vi "PostBuild.vi"(8 "error in (no error)":errorcluster, 9 "GeneratedFiles in":path[](array[path]), 10 "GeneratedDirectories in":path[](array[path]), 11 "Build in":refnum<class "AB_Build.lvclass">) -> (0 "error out":errorcluster, 1 "GeneratedFiles out":path[](array[path]), 2 "GeneratedDirectories out":path[](array[path]), 3 "Build out":refnum<class "AB_Build.lvclass">)   [LabVIEW 2020, in "AB_Build.lvclass"]
uses:
  <vilib>/AppBuilder/AB_Classes/Build/AB_Build.lvclass
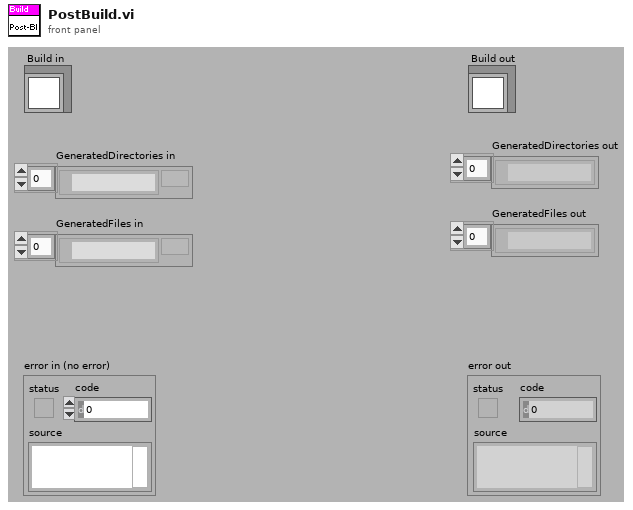
[diagram p1: front panel]
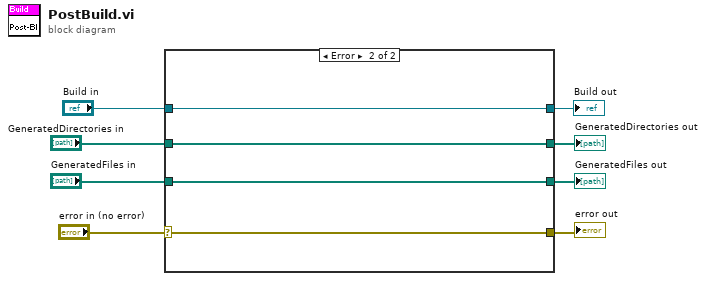
[diagram p0: block diagram]
diagram:
  n1 = case shown="Error" "error in (no error)" {
    selector: "error in (no error)" -> [w11 w16]
    tunnel: [w11 w16] -> w7
    tunnel: [w12 w15] -> w5
    tunnel: "Build in" -> [w12 w15]
    tunnel: [w10 w14] -> w4
    tunnel: "GeneratedDirectories in" -> [w10 w14]
    tunnel: [w9 w13] -> w2
    tunnel: "GeneratedFiles in" -> [w9 w13]
    frame No Error {
    }
    frame Error {
    }
  }
  "error out" <- w7
  "Build out" <- w5
  "GeneratedDirectories out" <- w4
  "GeneratedFiles out" <- w2
